vi "Read Output Values.vi"(7 "Unit Address (1)":u8=1, 8 "error in (no error)":errorcluster, 11 "VISA resource name":refnum<visa-resource-name>) -> (0 "error out":errorcluster, 1 "Manual Output Value":i32, 2 "Channel 1 Output Value":i32, 3 "VISA resource name out":refnum<visa-resource-name>, 4 "Feedforward Output Value":i32)   [LabVIEW 2014, in "Eurotherm 35xx Series.lvlib"]
doc: "This VI returns Output Values."
uses:
  <instrlib>/Eurotherm 35xx Series/Eurotherm 35xx Series.lvlib
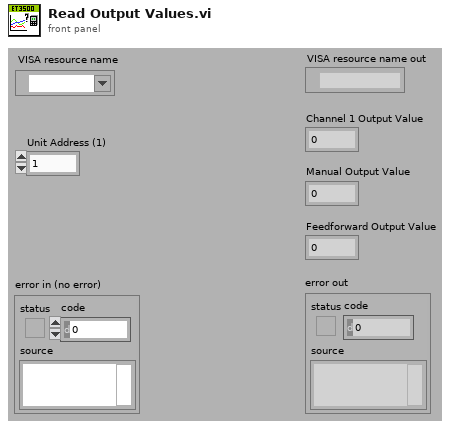
[diagram p1: front panel]
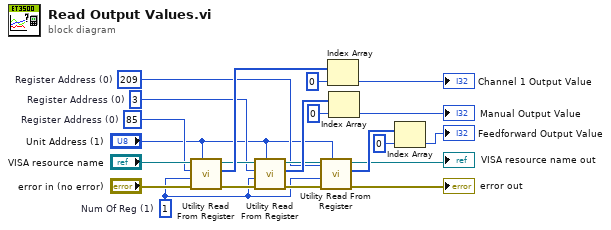
[diagram p0: block diagram]
diagram:
  w5 = 209  # Register Address (0)
  w6 = 3  # Register Address (0)
  w19 = 85  # Register Address (0)
  w9 = u16 1  # Num Of Reg (1)
  n1 = call <instrlib>:"Utility Read From Register.vi"("Unit Address (1)"="Unit Address (1)", "error in (no error)"="error in (no error)", "Num Of Reg (1)"=w9, "Register Address (0)"=w19, "VISA resource name"="VISA resource name") -> ("error out"=w10:errorcluster, "Data"=w20:i16[], "VISA resource name out"=w13:refnum<visa-resource-name>)  [unwired: 4 in]
  n2 = call <instrlib>:"Utility Read From Register.vi"("Unit Address (1)"="Unit Address (1)", "error in (no error)"=w10, "Num Of Reg (1)"=w9, "Register Address (0)"=w6, "VISA resource name"=w13) -> ("error out"=w11:errorcluster, "Data"=w16:i16[], "VISA resource name out"=w12:refnum<visa-resource-name>)  [unwired: 4 in]
  n3 = call <instrlib>:"Utility Read From Register.vi"("Unit Address (1)"="Unit Address (1)", "error in (no error)"=w11, "Num Of Reg (1)"=w9, "Register Address (0)"=w5, "VISA resource name"=w12) -> ("error out"=→"error out":errorcluster, "Data"=w15:i16[], "VISA resource name out"=→"VISA resource name out":refnum<visa-resource-name>)  [unwired: 4 in]
  n4 = Index Array(array=w20, index=0) -> (element=→"Channel 1 Output Value":i16)
  n5 = Index Array(array=w16, index=0) -> (element=→"Manual Output Value":i16)
  n6 = Index Array(array=w15, index=0) -> (element=→"Feedforward Output Value":i16)
